vi "Convert Shutdown Furnace to Heater State Enum-teardown.vi"(10 "Heater State":T1, 11 "test case ID":string) -> (3 "result":bool)   [LabVIEW 2018]
doc: "The teardown VI should be executed after the VI under test in the harness VI. In this VI you can evaluate the outputs of the VI under test.\n\nSee the Help Document for more information. (<b>Help</b> > <b>IncQuery Labs</b> > <b>InstaCoverage</b> > <b>InstaCoverage Help...</b>)"
uses:
  Libraries/Thermal Chamber Controller_DQMH/Heater State--enum.ctl
  Libraries/Thermal Chamber Controller_DQMH/Thermal Chamber Controller_DQMH.lvlib
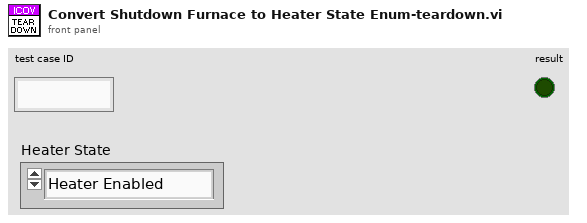
[diagram p1: front panel]
types:
  T1 = typedef "Thermal Chamber Controller_DQMH.lvlib/Heater State--enum.ctl" = enum16{"Heater Enabled", "Heater Disabled"}
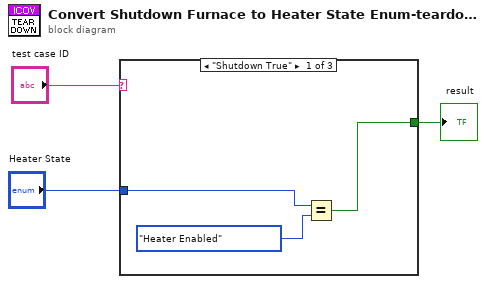
[diagram p0: block diagram]
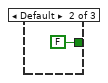
[diagram p2: hidden frame]
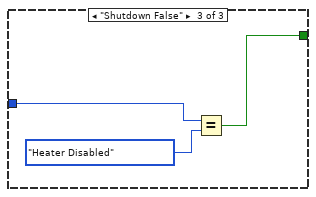
[diagram p3: hidden frame]
diagram:
  n1 = case shown="\"Shutdown True\"" "test case ID" {
    tunnel: [w4 FALSE w8] -> w2
    tunnel: "Heater State" -> [w6 _ w10]
    frame "Shutdown True" {
      n2 = Equal?(x=w6, y=Heater_State--enum."Heater Enabled" ("Heater State")) -> (x = y?=w4:bool)
    }
    frame Default {
    }
    frame "Shutdown False" {
      n3 = Equal?(x=w10, y=Heater_State--enum."Heater Disabled" ("Heater State")) -> (x = y?=w8:bool)
    }
  }
  "result" <- w2
